vi "Read States.vi"(8 "error in (no error)":errorcluster, 11 "GoAndKickTacticVSS in":refnum<class "GoAndKickTacticVSS.lvclass">) -> (0 "error out":errorcluster, 2 "States":enum16{"GoToBall", "Kick", "Exit"}(ring), 3 "GoAndKickTacticVSS out":refnum<class "GoAndKickTacticVSS.lvclass">)   [LabVIEW 2023, in "GoAndKickTacticVSS.lvclass"]
uses:
  GoAndKickTacticVSS.lvclass
  GoAndKickTacticVSS.lvclass/GoAndKickTacticVSS.ctl
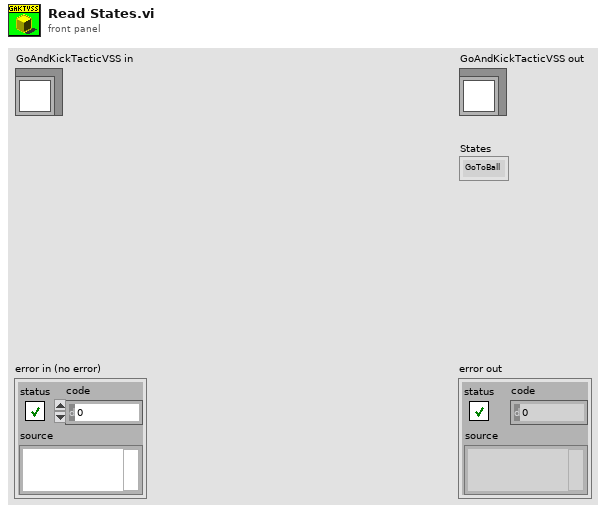
[diagram p1: front panel]
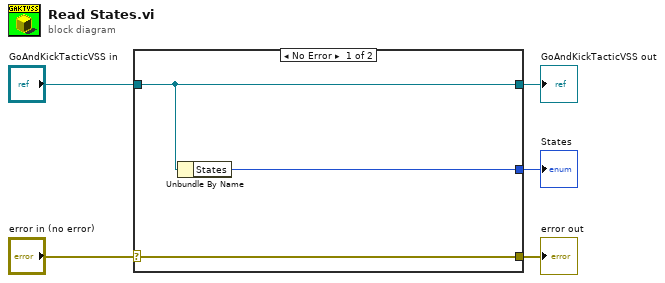
[diagram p0: block diagram]
diagram:
  n1 = case shown="No Error" "error in (no error)" {
    selector: "error in (no error)" -> [w8 w9]
    tunnel: [w8 w9] -> w4
    tunnel: [w7 w10] -> w2
    tunnel: "GoAndKickTacticVSS in" -> [w7 w10]
    tunnel: [w6 _] -> w1
    frame No Error {
      n2 = Unbundle By Name(w7) -> ("States"=w6:enum16{"GoToBall", "Kick", "Exit"})
    }
    frame Error {
    }
  }
  "error out" <- w4
  "GoAndKickTacticVSS out" <- w2
  "States" <- w1
